vi "VI Panel Origin.vi"(8 "error in (no error)":errorcluster, 10 "Origin":T1, 11 "This VI":refnum<vi>) -> (0 "error out":errorcluster)   [LabVIEW 2023, in "GUI.lvlib" / "Vitesco Launcher.lvlib"]
uses:
  Vitesco Launcher.lvlib
  <vilib>/Utility/miscctls.llb/LVPointTypeDef.ctl
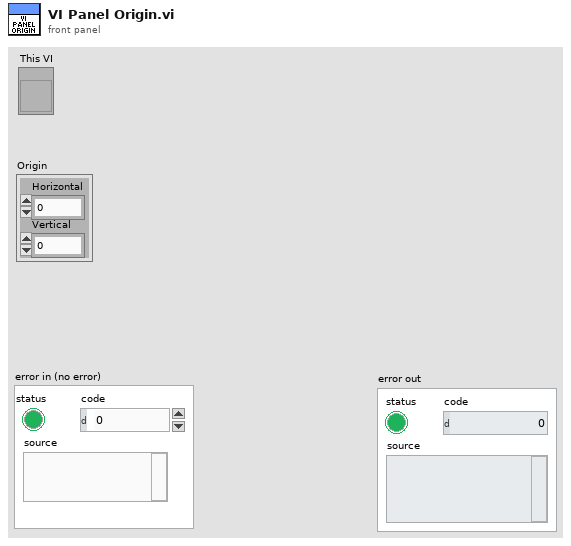
[diagram p1: front panel]
types:
  T1 = typedef "LVPointTypeDef.ctl" = cluster{"Horizontal":i16, "Vertical":i16}
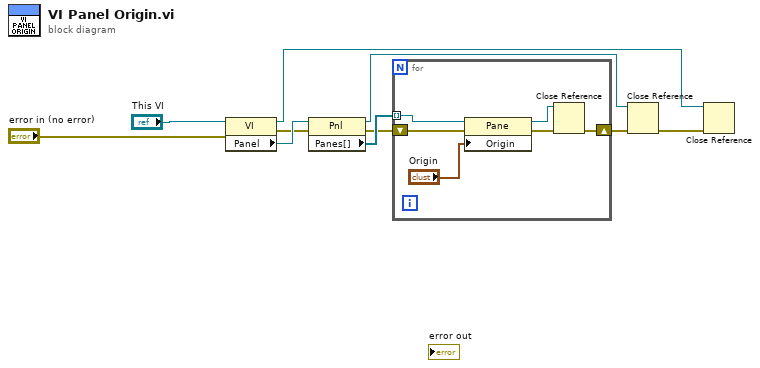
[diagram p0: block diagram]
diagram:
  n1 = property class="VI"(reference="This VI", error in="error in (no error)") -> (reference out=w3:refnum<vi>, error out=w9:errorcluster, "Panel"=w10:refnum<vi>)
  n2 = property class="Pnl"(reference=w10, error in=w9) -> (reference out=w4:refnum<vi>, error out=w7:errorcluster, "Panes[]"=w8:refnum<vi>[])
  n3 = for {
    tunnel: w8 -> [w16] mode=indexing
    shift-right: [w12] -> w6
    shift-left: w7 -> [w15]
    n4 = property class="Pane"(reference=w16, error in=w15, "Origin"="Origin") -> (reference out=w11:refnum<vi>, error out=w14:errorcluster)
    n5 = Close Reference(reference=w11, error in (no error)=w14) -> (error out=w12:errorcluster)
  }
  n6 = Close Reference(reference=w4, error in (no error)=w6) -> (error out=w5:errorcluster)
  n7 = Close Reference(reference=w3, error in (no error)=w5) -> ()  [unwired: 1 out]
